vi "Get_No_Top_Level_Message.vi"(11 "Build in":refnum<class "AB_DLL.lvclass">) -> (2 "No top level VI":string, 3 "Build out":refnum<class "AB_DLL.lvclass">)   [LabVIEW 2020, in "AB_DLL.lvclass"]
uses:
  <vilib>/AppBuilder/AB_Classes/DLL/AB_DLL.lvclass
  <vilib>/AppBuilder/AB_Classes/DLL/AB_DLL.lvclass/AB_DLL.ctl
  <resource>/Framework/Providers/Common/provcom_StringGlobals.vi
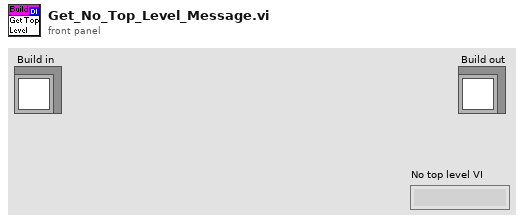
[diagram p1: front panel]
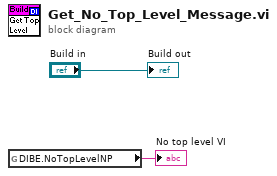
[diagram p0: block diagram]
diagram:
  n1 = global read "provcom_StringGlobals.vi" "DIBE.NoTopLevelNP"() -> (→"No top level VI":string)
  "Build out" <- "Build in"
